vi "main screen queue out Unitest.vi"(8 "error in (no error)":errorcluster) -> (0 "error out":errorcluster)   [LabVIEW 2025]
uses:
  REF Enum Unitest.ctl
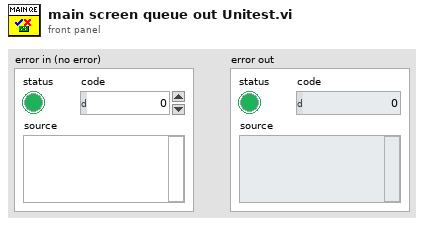
[diagram p1: front panel]
types:
  T1 = typedef "REF Enum Unitest.ctl" = enum16{"Init", "UI Loop", "LOAD COM LOOP", "HEAVE MOTOR COM LOOP", "SWAY MOTOR COM LOOP", "RAMP MOTOR COM LOOP", "TEMPERATURE COM LOOP", "HUMIDITY COM PORT", "ECR PORT", "MONITOR LOOP", "PROGRAM LOOP", "LOAD PID", "REPORT", "ACOUSTIC"}
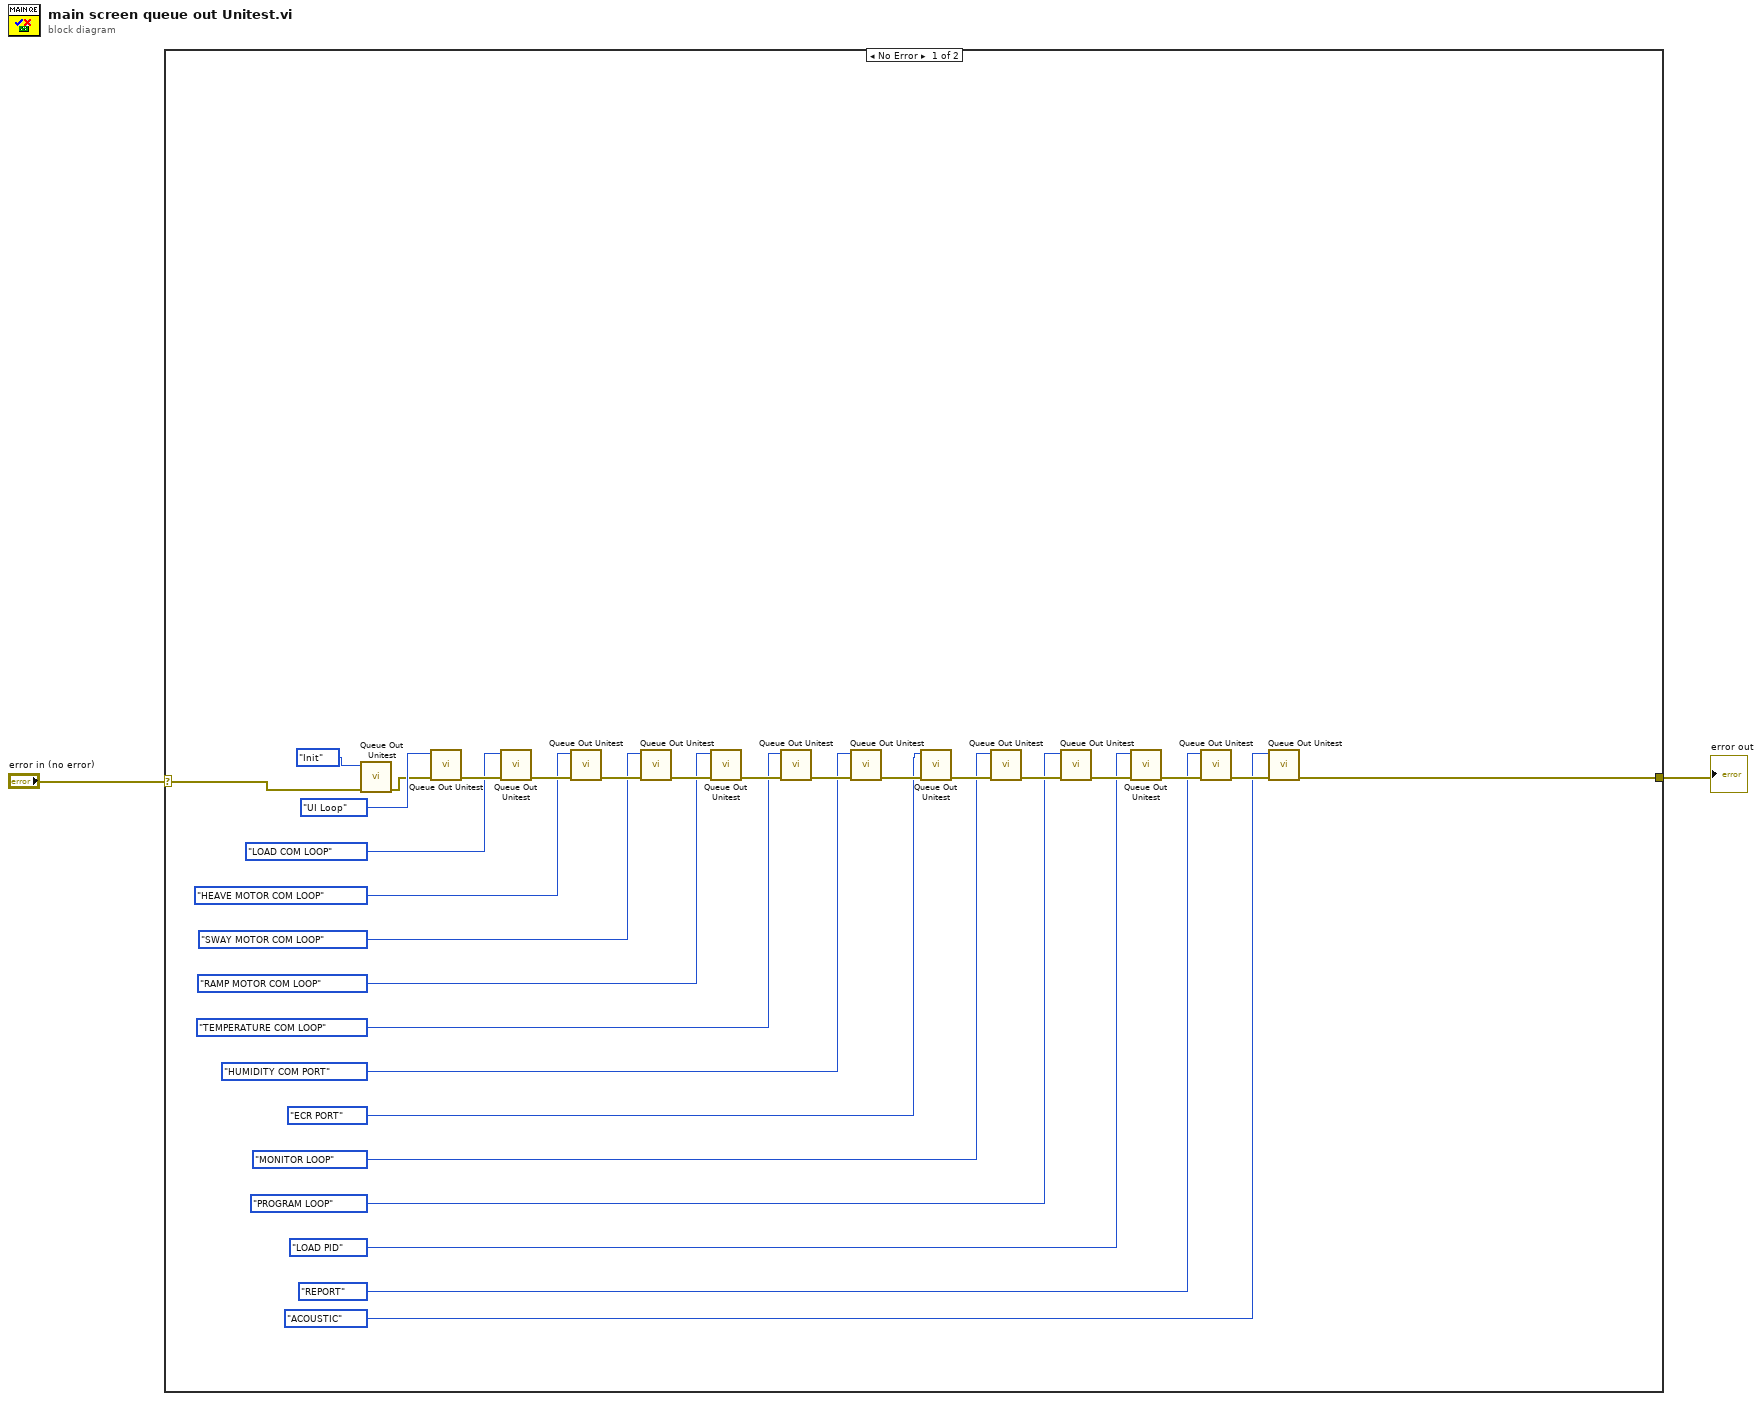
[diagram p0: block diagram]
diagram:
  n1 = case shown="No Error" "error in (no error)" {
    selector: "error in (no error)" -> [w31 _]
    tunnel: [w4 _] -> w2
    frame No Error {
      n2 = call "Queue Out Unitest.vi"("error in"=w31, 11:REF_Enum_Unitest."Init") -> ("error out"=w28:errorcluster)  [unwired: 9 in]
      n3 = call "Queue Out Unitest.vi"("error in"=w28, 11:REF_Enum_Unitest."UI Loop") -> ("error out"=w27:errorcluster)  [unwired: 9 in]
      n4 = call "Queue Out Unitest.vi"("error in"=w27, 11:REF_Enum_Unitest."LOAD COM LOOP") -> ("error out"=w26:errorcluster)  [unwired: 9 in]
      n5 = call "Queue Out Unitest.vi"("error in"=w26, 11:REF_Enum_Unitest."HEAVE MOTOR COM LOOP") -> ("error out"=w25:errorcluster)  [unwired: 9 in]
      n6 = call "Queue Out Unitest.vi"("error in"=w25, 11:REF_Enum_Unitest."SWAY MOTOR COM LOOP") -> ("error out"=w24:errorcluster)  [unwired: 9 in]
      n7 = call "Queue Out Unitest.vi"("error in"=w24, 11:REF_Enum_Unitest."RAMP MOTOR COM LOOP") -> ("error out"=w23:errorcluster)  [unwired: 9 in]
      n8 = call "Queue Out Unitest.vi"("error in"=w23, 11:REF_Enum_Unitest."TEMPERATURE COM LOOP") -> ("error out"=w22:errorcluster)  [unwired: 9 in]
      n9 = call "Queue Out Unitest.vi"("error in"=w22, 11:REF_Enum_Unitest."HUMIDITY COM PORT") -> ("error out"=w21:errorcluster)  [unwired: 9 in]
      n10 = call "Queue Out Unitest.vi"("error in"=w21, 11:REF_Enum_Unitest."ECR PORT") -> ("error out"=w20:errorcluster)  [unwired: 9 in]
      n11 = call "Queue Out Unitest.vi"("error in"=w20, 11:REF_Enum_Unitest."MONITOR LOOP") -> ("error out"=w19:errorcluster)  [unwired: 9 in]
      n12 = call "Queue Out Unitest.vi"("error in"=w19, 11:REF_Enum_Unitest."PROGRAM LOOP") -> ("error out"=w18:errorcluster)  [unwired: 9 in]
      n13 = call "Queue Out Unitest.vi"("error in"=w18, 11:REF_Enum_Unitest."LOAD PID") -> ("error out"=w17:errorcluster)  [unwired: 9 in]
      n14 = call "Queue Out Unitest.vi"("error in"=w17, 11:REF_Enum_Unitest."REPORT") -> ("error out"=w5:errorcluster)  [unwired: 9 in]
      n15 = call "Queue Out Unitest.vi"("error in"=w5, 11:REF_Enum_Unitest."ACOUSTIC") -> ("error out"=w4:errorcluster)  [unwired: 9 in]
    }
    frame Error {
    }
  }
  "error out" <- w2
